vi "Convert Date to Timestamp.vi"(2 "Date":T1) -> (7 "Time Stamp":timestamp)   [LabVIEW 2021, in "Time.lvlib"]
uses:
  Time.lvlib
  PicoStart Date.ctl
  <vilib>/Utility/miscctls.llb/LVDateTimeRec.ctl
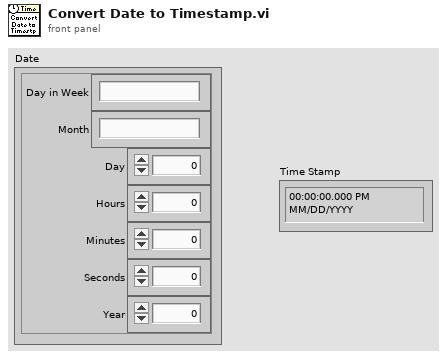
[diagram p1: front panel]
types:
  T1 = typedef "Time.lvlib/PicoStart Date.ctl" = cluster{"Day in Week":string, "Month":string, "Day":i32, "Hours":i32, "Minutes":i32, "Seconds":i32, "Year":i32}
  T2 = typedef "LVDateTimeRec.ctl" = cluster{"fractional second":dbl, "second":i32, "minute":i32, "hour":i32, "day of month":i32, "month":i32, "year":i32, "day of week":i32, "day of year":i32, "DST":i32}
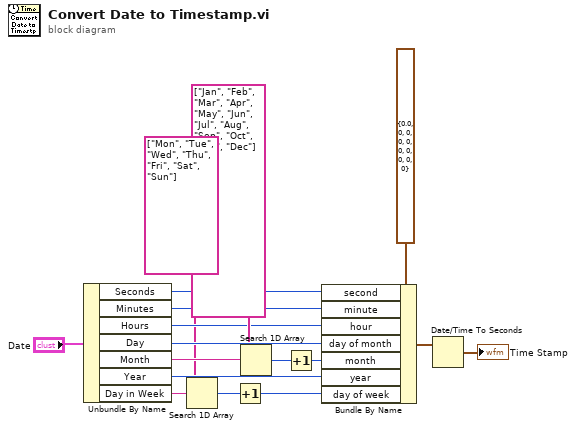
[diagram p0: block diagram]
diagram:
  n1 = Unbundle By Name("Date") -> ("Seconds"=w8:i32, "Minutes"=w7:i32, "Hours"=w6:i32, "Day"=w14:i32, "Month"=w13:string, "Year"=w9:i32, "Day in Week"=w5:string)
  n2 = Search 1D Array(1D array=string[] ["Mon", "Tue", "Wed", "Thu", "Fri", "Sat", "Sun"], element=w5) -> (index of element=w4:i32)  [unwired: 1 in]
  n3 = Increment(x=w4) -> (x+1=w3:i32)
  n4 = Search 1D Array(1D array=string[] ["Jan", "Feb", "Mar", "Apr", "May", "Jun", "Jul", "Aug", "Sep", "Oct", "Nov", "Dec"], element=w13) -> (index of element=w12:i32)  [unwired: 1 in]
  n5 = Increment(x=w12) -> (x+1=w10:i32)
  n6 = Bundle By Name(cluster=T2 {"fractional second"=0.0, "second"=0, "minute"=0, "hour"=0, "day of month"=0, "month"=0, "year"=0, "day of week"=0, "day of year"=0, "DST"=0} ("date time rec"), "second"=w8, "minute"=w7, "hour"=w6, "day of month"=w14, "month"=w10, "year"=w9, "day of week"=w3) -> (w17:T2)
  n7 = Date/Time To Seconds(2:w17) -> (0:→"Time Stamp":timestamp)  [unwired: 1 in]
